vi "Handle Error.vi"(8 "error in (no error)":errorcluster, 11 "TCP Receive in":refnum<class "TCP Receive.lvclass">) -> (0 "error out":errorcluster, 3 "TCP Receive out":refnum<class "TCP Receive.lvclass">)   [LabVIEW 2020, in "TCP Receive.lvclass"]
uses:
  TCP Receive.lvclass
  C:/Program Files (x86)/National Instruments/LabVIEW 2020/vi.lib/addons/_Workers/Library/Classes/Worker/Worker.lvclass
  TCP Receive.lvclass/TCP Receive.ctl
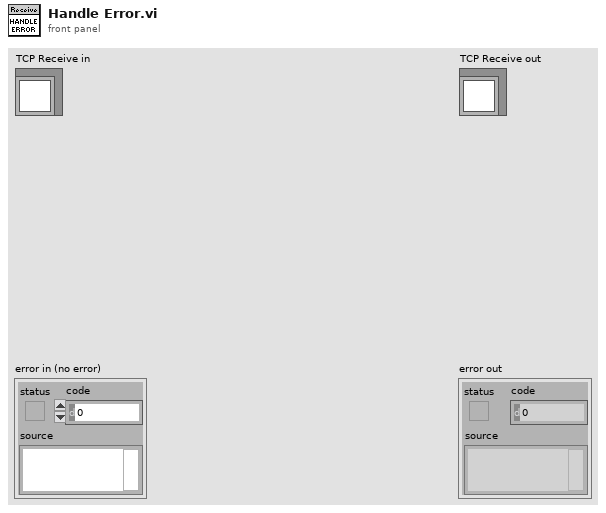
[diagram p1: front panel]
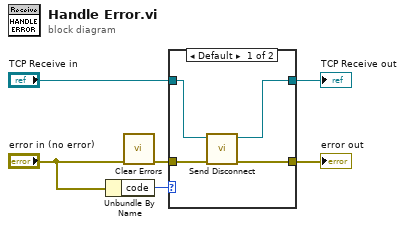
[diagram p0: block diagram]
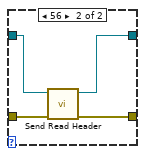
[diagram p2: hidden frame]
diagram:
  n1 = Unbundle By Name("error in (no error)") -> ("code"=w6:i32)
  n2 = call <vilib>:"Clear Errors.vi"("error in (no error)"="error in (no error)") -> ("error out"=w1:errorcluster)  [unwired: 5 in, 1 out]
  n3 = case shown="Default" w6 {
    tunnel: w1 -> [w10 w14]
    tunnel: "TCP Receive in" -> [w8 w12]
    tunnel: [w9 w13] -> w2
    tunnel: [w7 w11] -> w4
    frame Default {
      n4 = call "Send Disconnect.vi"("error in (no error)"=w10, "TCP Receive in"=w8) -> ("error out"=w9:errorcluster, "TCP Receive out"=w7:refnum<class "TCP Receive.lvclass">)  [unwired: 8 in]
    }
    frame 56 {
      n5 = call "Send Read Header.vi"("error in (no error)"=w14, "TCP Receive in"=w12) -> ("error out"=w13:errorcluster, "TCP Receive out"=w11:refnum<class "TCP Receive.lvclass">)  [unwired: 8 in]
    }
  }
  "error out" <- w2
  "TCP Receive out" <- w4
